vi "Recibo-Varaint.vi"() -> ()   [LabVIEW 2016]
panel:
  out "values 3":dbl
  out "values 2":i8
  out "data":string
  out "values":bool
  in  "Detener":bool
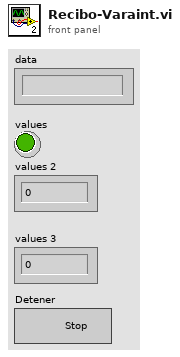
[diagram p1: front panel]
types:
  T1 = enum16{"Read", "Write", "ReadWrite", "BufferedRead", "BufferedReadWrite"}
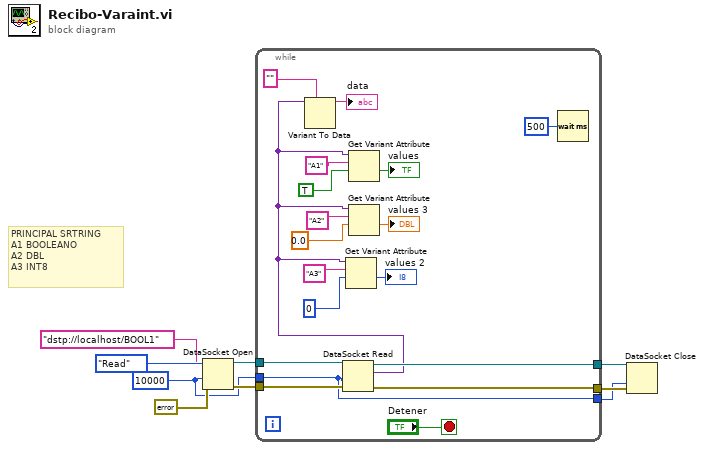
[diagram p0: block diagram]
diagram:
  w2 = 10000 ("ms timeout (10000)")
  # "PRINCIPAL SRTRING \nA1 BOOLEANO\nA2 DBL\nA3 INT8"
  n1 = DataSocket Open(8:errorcluster {"status"=FALSE, "code"=0, "source"=""} ("error in (no error)"), 9:w2, 10:T1."Read" ("mode"), 11:"dstp://localhost/BOOL1" ("connection in")) -> (0:w6:errorcluster, 3:w7:refnum<k13>)
  n2 = while {
    tunnel: w6 -> [w26]
    tunnel: w7 -> [w25]
    tunnel: [w24] -> w8
    tunnel: [w23] -> w9
    tunnel: w2 -> [w22]
    tunnel: [w22] -> w1
    stop <- "Detener" stop-if-true
    n3 = DataSocket Read(8:w26, 9:w22, 11:w25) -> (0:w23:errorcluster, 2:w10:variant, 3:w24:refnum<k13>)  [unwired: 2 in, 4 out]
    n4 = Variant To Data(type="", Variant=w10) -> (data=→"data":string)  [unwired: 1 in, 1 out]
    n5 = Get Variant Attribute(Variant=w10, name="A3", default value (empty Variant)=i8 0) -> (value=→"values 2":i8)  [unwired: 1 in, 3 out]
    n6 = Get Variant Attribute(Variant=w10, name="A1", default value (empty Variant)=TRUE) -> (value=→"values":bool)  [unwired: 1 in, 3 out]
    n7 = Get Variant Attribute(Variant=w10, name="A2", default value (empty Variant)=0.0) -> (value=→"values 3":dbl)  [unwired: 1 in, 3 out]
    n8 = Wait (ms)(milliseconds to wait=u32 500) -> ()  [unwired: 1 out]
  }
  n9 = DataSocket Close(8:w9, 9:w1, 11:w8) -> ()  [unwired: 2 out]
